vi "Test 1.vi"() -> ()   [LabVIEW 2023]
panel:
  in  "Bayer::Pattern":u32(ring)=5 items=["Use hardware value"=5, "None"=0, "GB"=1, "GR"=2, "BG"=3, "RG"=4]
  in  "Bayer::Gain R":dbl=1.0 min=0.0 max=3.999
  in  "Bayer::Gain G":dbl=1.0 min=0.0 max=3.999
  in  "Bayer::Gain B":dbl=1.0 min=0.0 max=3.999
  in  "Bayer::Algorithm":u32(ring) items=["Bilinear", "VNG"]
  out "error out":errorcluster
  out "Frame Rate":dbl
  out "Image Number":u32
  in  "Sharpness::Value":i64=2 min=0 max=7 step=1
  in  "Saturation::Value":i64=64 min=0 max=100 step=1
  in  "error in":errorcluster
  in  "Hue::Value":dbl min=-1.8 max=1.8
  in  "Gamma::Value":dbl=1.2 min=0.9 max=1.5
  in  "Gain::Value":i64=4 min=4 max=8 step=1
  in  "Contrast::Value":dbl=0.32 min=0.0 max=2.55
  in  "Brightness::Value":i64=100 min=0 max=255 step=1
  in  "Backlight Compensation::Mode":u32(ring)=2 items=["Manual"=2]
  in  "Stop (F)":bool
  out "Image Out":T1(plugin-control)
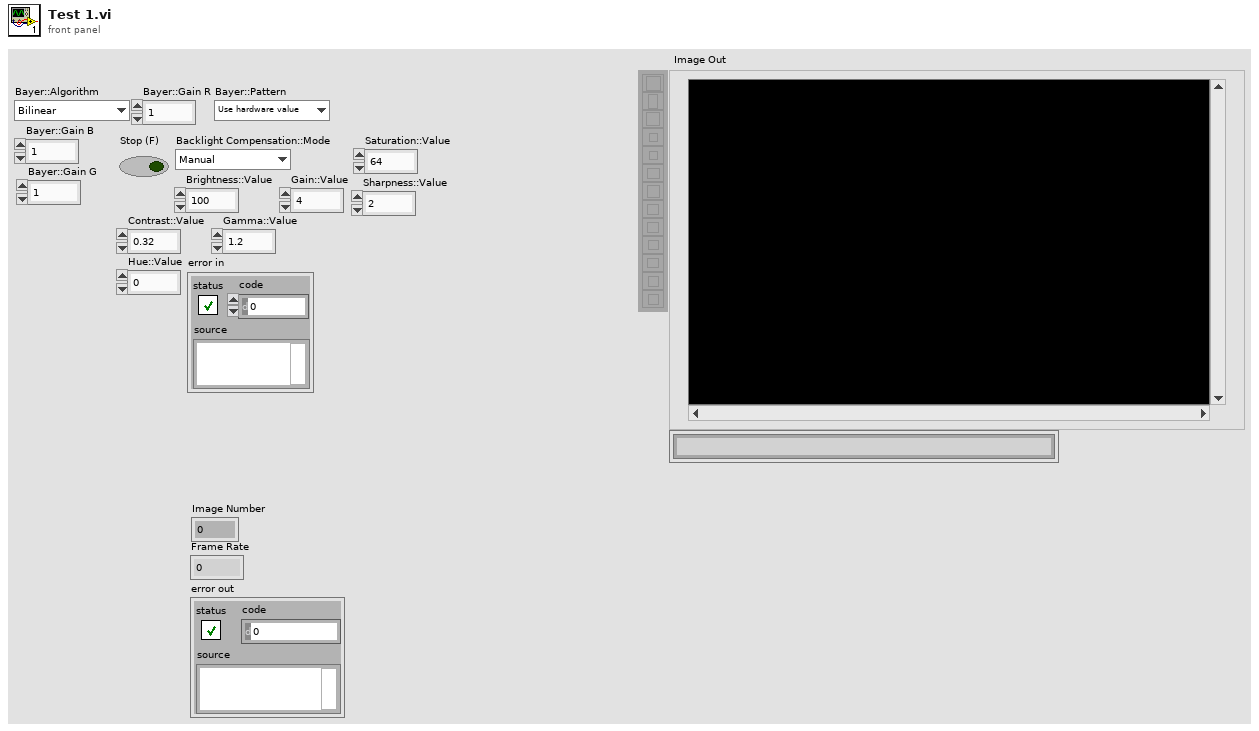
[diagram p1: front panel]
types:
  T1 = typedef "IMAQ Image.ctl" = refnum<image>
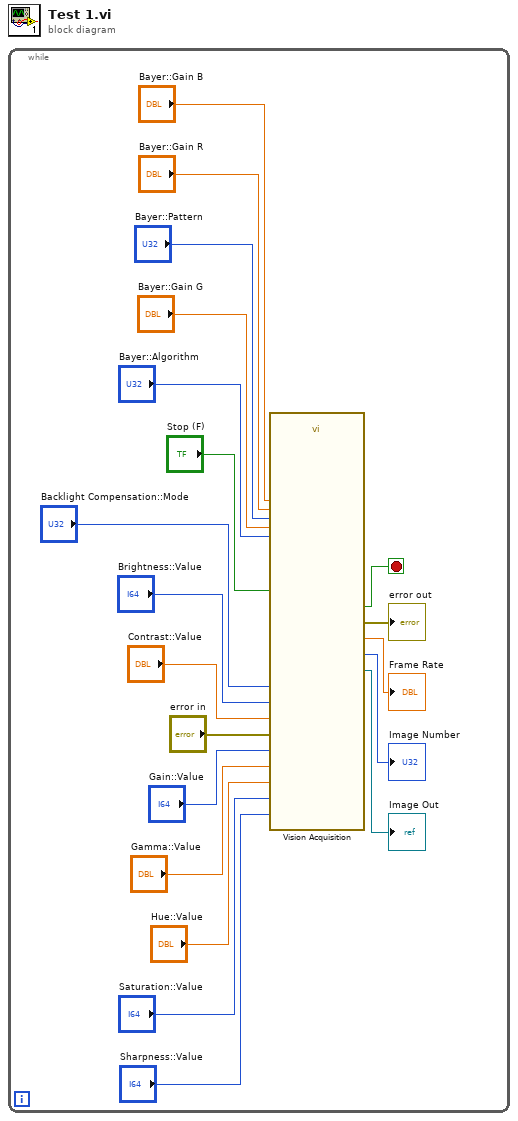
[diagram p0: block diagram]
diagram:
  n1 = while {
    stop <- w18 stop-if-true
    n2 = call "Vision Acquisition"("Backlight Compensation::Mode"="Backlight Compensation::Mode", "Brightness::Value"="Brightness::Value", "Contrast::Value"="Contrast::Value", "Gain::Value"="Gain::Value", "Gamma::Value"="Gamma::Value", "Stop (F)"="Stop (F)", "Hue::Value"="Hue::Value", "error in"="error in", "Saturation::Value"="Saturation::Value", "Sharpness::Value"="Sharpness::Value", "Bayer::Algorithm"="Bayer::Algorithm", "Bayer::Gain B"="Bayer::Gain B", "Bayer::Gain G"="Bayer::Gain G", "Bayer::Gain R"="Bayer::Gain R", "Bayer::Pattern"="Bayer::Pattern") -> ("Image Out"=→"Image Out":T1, "Image Number"=→"Image Number":u32, "Frame Rate"=→"Frame Rate":dbl, "Stopped"=w18:bool, "error out"=→"error out":errorcluster)  [unwired: 8 in]
  }
